vi "Create Event1.vi"() -> (3 "Event Out":T1)   [LabVIEW 2015]
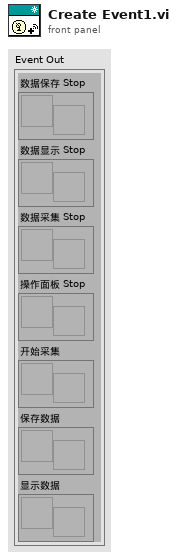
[diagram p1: front panel]
types:
  T1 = cluster{"数据保存 Stop":refnum<user-event>, "数据显示 Stop":refnum<user-event>, "数据采集 Stop":refnum<user-event>, "操作面板 Stop":refnum<user-event>, "开始采集":refnum<user-event>, "保存数据":refnum<user-event>, "显示数据":refnum<user-event>}
  T2 = cluster{"数据保存 Stop":refnum<user-event>, "数据显示 Stop":refnum<user-event>, "数据采集 Stop":refnum<user-event>, "操作面板 Stop":refnum<user-event>, "开始采集":refnum<user-event>, "显示数据":refnum<user-event>, "保存数据":refnum<user-event>}
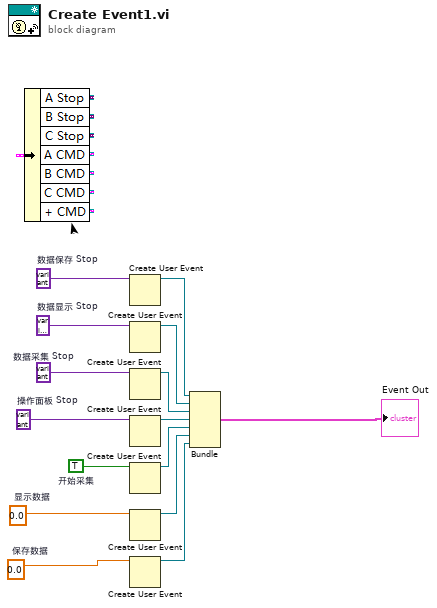
[diagram p0: block diagram]
diagram:
  w1 = 0.0  # 保存数据
  w2 = 0.0  # 显示数据
  w4 = TRUE  # 开始采集
  w6 = variant  # 操作面板 Stop
  w13 = variant  # 数据采集 Stop
  w14 = variant  # 数据显示 Stop
  w15 = variant  # 数据保存 Stop
  n1 = Create User Event(user event datatype=w15) -> (user event=w12:refnum<user-event>)  [unwired: 1 in, 1 out]
  n2 = Create User Event(user event datatype=w14) -> (user event=w11:refnum<user-event>)  [unwired: 1 in, 1 out]
  n3 = Create User Event(user event datatype=w13) -> (user event=w10:refnum<user-event>)  [unwired: 1 in, 1 out]
  n4 = Create User Event(user event datatype=w6) -> (user event=w5:refnum<user-event>)  [unwired: 1 in, 1 out]
  n5 = Create User Event(user event datatype=w4) -> (user event=w9:refnum<user-event>)  [unwired: 1 in, 1 out]
  n6 = Create User Event(user event datatype=w2) -> (user event=w8:refnum<user-event>)  [unwired: 1 in, 1 out]
  n7 = Create User Event(user event datatype=w1) -> (user event=w7:refnum<user-event>)  [unwired: 1 in, 1 out]
  n8 = Bundle("数据保存 Stop"=w12, "数据显示 Stop"=w11, "数据采集 Stop"=w10, "操作面板 Stop"=w5, "开始采集"=w9, "显示数据"=w8, "保存数据"=w7) -> (→"Event Out":T2)  [unwired: 1 in]
